vi "GetAlarms.vi"(0 "NeedleValve in":refnum<class "NeedleValve.lvclass">, 11 "error in (no error)":errorcluster) -> (4 "NeedleValve out":refnum<class "NeedleValve.lvclass">, 6 "Alarm":bool, 8 "Warning":bool, 15 "error out":errorcluster)   [LabVIEW 2019, in "NeedleValve.lvclass"]
uses:
  NeedleValve.lvclass
  NeedleValve.lvclass/NeedleValve.ctl
  DA_class/DA.lvclass
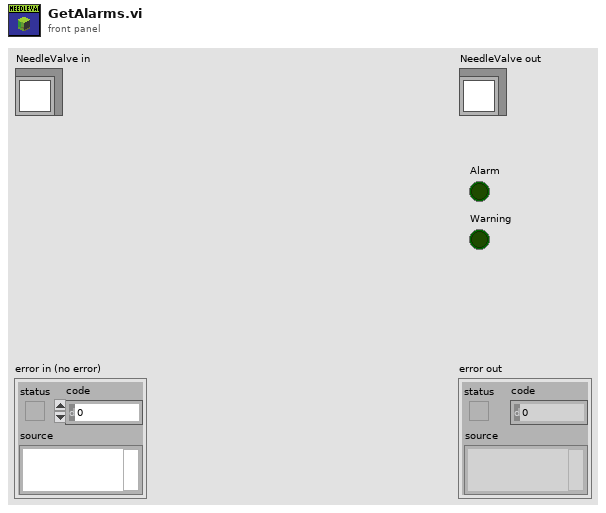
[diagram p1: front panel]
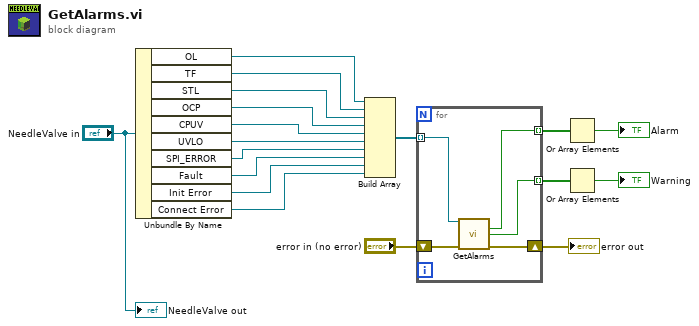
[diagram p0: block diagram]
diagram:
  n1 = Unbundle By Name("NeedleValve in") -> ("OL"=w18:refnum<class "DA.lvclass">, "TF"=w11:refnum<class "DA.lvclass">, "STL"=w10:refnum<class "DA.lvclass">, "OCP"=w9:refnum<class "DA.lvclass">, "CPUV"=w8:refnum<class "DA.lvclass">, "UVLO"=w7:refnum<class "DA.lvclass">, "SPI_ERROR"=w6:refnum<class "DA.lvclass">, "Fault"=w5:refnum<class "DA.lvclass">, "Init Error"=w4:refnum<class "DA.lvclass">, "Connect Error"=w1:refnum<class "DA.lvclass">)
  n2 = Build Array(w18, w11, w10, w9, w8, w7, w6, w5, w4, w1) -> (w17:refnum<class "DA.lvclass">[])
  n3 = for {
    tunnel: w17 -> [w23] mode=indexing
    tunnel: [w22] -> w16 mode=indexing
    tunnel: [w21] -> w15 mode=indexing
    shift-right: [w20] -> w13
    shift-left: "error in (no error)" -> [w19]
    n4 = call-dynamic "GetAlarms.vi"("DA in"=w23, "error in (no error)"=w19) -> ("Alarm"=w22:bool, "Warning"=w21:bool, "error out"=w20:errorcluster)  [unwired: 10 in, 1 out]
  }
  "error out" <- w13
  n5 = Or Array Elements(Boolean array=w16) -> (logical OR=→"Alarm":bool)
  n6 = Or Array Elements(Boolean array=w15) -> (logical OR=→"Warning":bool)
  "NeedleValve out" <- "NeedleValve in"
